vi "LOG Build MSG Data.vi"(1 "Message":string="Update", 8 "Replace":bool) -> (15 "MSG data":variant)   [LabVIEW 2020, in "LOG.lvlib"]
uses:
  LOG.lvlib
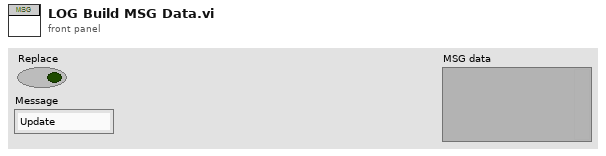
[diagram p1: front panel]
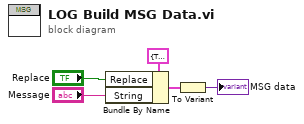
[diagram p0: block diagram]
diagram:
  n1 = Bundle By Name(cluster=cluster{"Replace":bool, "String":string} {"Replace"=TRUE, "String"="1"}, "Replace"="Replace", "String"="Message") -> (w2:cluster{"Replace":bool, "String":string})
  n2 = To Variant(anything=w2) -> (Variant=→"MSG data":variant)
